vi "puta que pariu.vi"() -> ()   [LabVIEW 2022 SP3]
uses:
  <vilib>/ActorFramework/Actor/Actor.lvclass
  Vision Receiver/Vision Receiver/Vision Receiver.lvclass
  C:/Program Files (x86)/National Instruments/LabVIEW 2022/vi.lib/MGI/Monitored Actor/Monitored Actor/Monitored Actor/Monitored Actor.lvclass
  C:/Program Files (x86)/National Instruments/LabVIEW 2022/vi.lib/ActorFramework/Actor/Actor.lvclass
  C:/Users/ebert/Documents/codes/ssl/repo/Phoenix Reborn/Vision Receiver/Vision Receiver/Vision Receiver.lvclass
  C:/Users/ebert/Documents/codes/ssl/repo/Phoenix Reborn/UDP Data Receiver/UDP Data Receiver/UDP Data Receiver.lvclass
  Vision.lvclass
  C:/Users/ebert/Documents/codes/ssl/repo/Phoenix Reborn/Vision/Vision/Vision.lvclass
panel:
  in  "Vision in":refnum<class "Vision.lvclass">
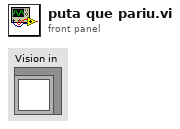
[diagram p1: front panel]
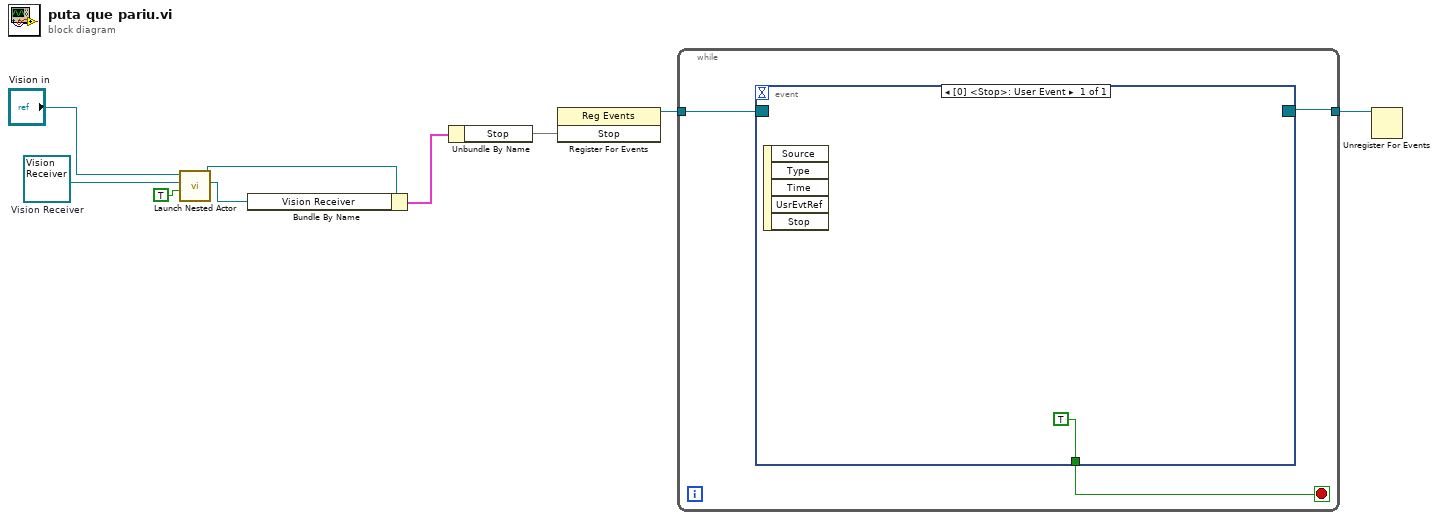
[diagram p0: block diagram]
diagram:
  w6 = refnum<class "Vision Receiver.lvclass"> refnum  # Vision Receiver
  n1 = call <vilib>:"Launch Nested Actor.vi"("Auto-stop? (T)"=TRUE, "Nested Actor"=w6, "Caller Actor in"="Vision in") -> ("Nested Actor's Enqueuer"=w4:refnum<class "Message Enqueuer.lvclass">, "Caller Actor out"=w3:refnum<class "Vision.lvclass">)  [unwired: 6 in, 1 out]
  n2 = Bundle By Name(cluster=w3, "Vision Receiver"=w4) -> (w2:cluster{})
  n3 = Unbundle By Name(w2) -> ("Stop"=w9)
  n4 = register-events(w9) -> (reference out=w8:refnum<event-registration>)  [unwired: 2 in, 1 out]
  n5 = while {
    tunnel: w8 -> [w12]
    tunnel: [w11] -> w7
    stop <- w10 stop-if-true
    n6 = event shown="[0] <Stop>: User Event" {
      selector: w12 -> [_]
      dyn-events: [_] -> w11
      timeout: _ -> [_]
      tunnel: [TRUE] -> w10
      event User Event {
        n7 = event-data() -> ()  [unwired: 1 in, 5 out]
      }
    }
  }
  n8 = Unregister For Events(event registration refnum=w7) -> ()  [unwired: 1 in, 1 out]
